vi "ControlPlans.vi"(8 "error in (no error)":errorcluster, 11 "ByteGSAPIBase in":refnum<class "ByteGSAPIBase.lvclass">) -> (0 "error out":errorcluster, 2 "Values":T1[](array[typedef]), 3 "ByteGSAPIBase out":refnum<class "ByteGSAPIBase.lvclass">)   [LabVIEW 2019, in "ByteGSWebAPI.lvlib" / "ByteGSAPIBase.lvclass"]
uses:
  ByteGSAPIBase.lvclass
  ControlPlan.ctl
  ByteGSAPIBase.lvclass/ByteGSAPIBase.ctl
  <vilib>/Bytelabs/ByteREST/ByteRESTClass/ByteRESTBase/RESTBase.lvclass
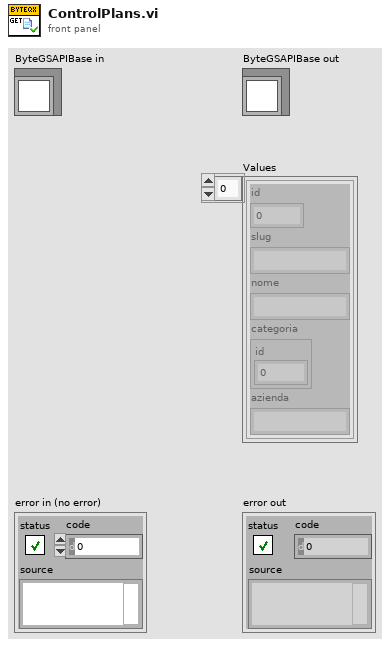
[diagram p1: front panel]
types:
  T1 = typedef "ByteGSWebAPI.lvlib/ByteGSAPIBase.lvclass/ControlPlan.ctl" = cluster{"id":i32, "slug":string, "nome":string, "categoria":cluster{"id":i32}, "azienda":string}
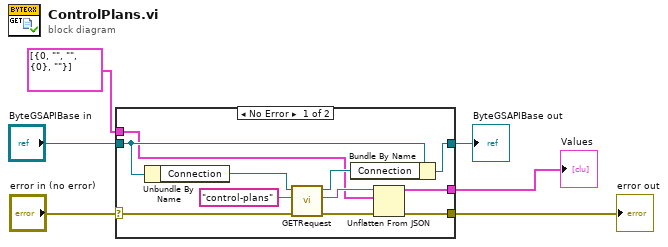
[diagram p0: block diagram]
diagram:
  n1 = case shown="No Error" "error in (no error)" {
    selector: "error in (no error)" -> [w8 w20]
    tunnel: [w7 w20] -> w3
    tunnel: T1[] [{"id"=0, "slug"="", "nome"="", "categoria"={"id"=0}, "azienda"=""}] -> [w10 w19]
    tunnel: [w9 w19] -> w1
    tunnel: [w14 w18] -> w4
    tunnel: "ByteGSAPIBase in" -> [w17 w18]
    frame No Error {
      n2 = Unbundle By Name(w17) -> ("Connection"=w16:refnum<class "RESTBase.lvclass">)
      n3 = call-dynamic "GETRequest.vi"("error in (no error)"=w8, "Request"="control-plans", "ByteRESTBase in"=w16) -> ("error out"=w15:errorcluster, "Body"=w11:string, "ByteRESTBase out"=w13:refnum<class "RESTBase.lvclass">)  [unwired: 5 in, 1 out]
      n4 = Bundle By Name(cluster=w17, "Connection"=w13) -> (w14:refnum<class "ByteGSAPIBase.lvclass">)
      n5 = Unflatten From JSON(JSON string=w11, type and defaults=w10, error in (no error)=w15) -> (value=w9:T1[], error out=w7:errorcluster)  [unwired: 4 in]
    }
    frame Error {
    }
  }
  "error out" <- w3
  "ByteGSAPIBase out" <- w4
  "Values" <- w1
